vi "Set Server Certificate File.vi"(10 "Server Certificate File (.crt)":path, 11 "OOP Server in":refnum<class "TestDataMarshal.lvclass">) -> (3 "OOP Server out":refnum<class "TestDataMarshal.lvclass">)   [LabVIEW 2019, in "TestDataMarshal.lvlib" / "TestDataMarshal.lvclass"]
uses:
  TestDataMarshal.lvclass
  TestDataMarshal.lvclass/TestDataMarshal.ctl
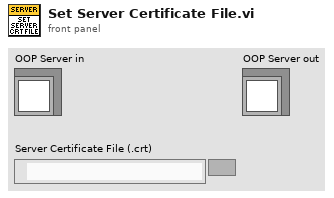
[diagram p1: front panel]
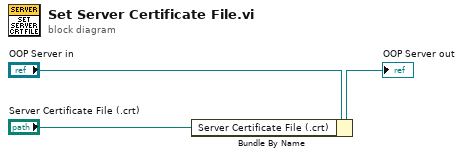
[diagram p0: block diagram]
diagram:
  n1 = Bundle By Name(cluster="OOP Server in", "Server Certificate File (.crt)"="Server Certificate File (.crt)") -> (→"OOP Server out":refnum<class "TestDataMarshal.lvclass">)
